vi "LS218_READ_KELVIN.vi"(3 "entrée d'erreur (pas d'erreur)":errorcluster, 4 "numéro voie":i32, 5 "Refnum VISA en entrée":refnum<visa-resource-name>) -> (0 "sortie d'erreur":errorcluster, 1 "T_Kelvin":dbl, 2 "Nom de ressource VISA en sortie":refnum<visa-resource-name>)   [LabVIEW 2016]
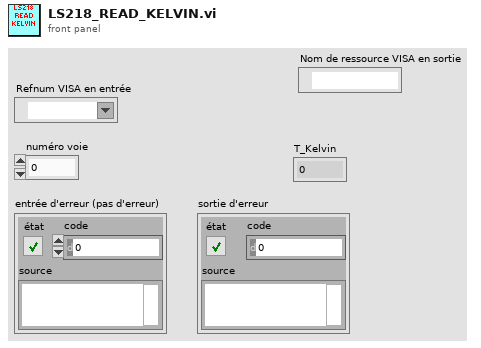
[diagram p1: front panel]
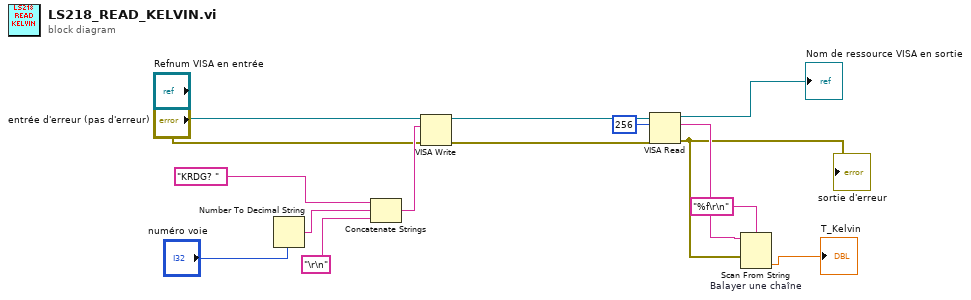
[diagram p0: block diagram]
diagram:
  n1 = Number To Decimal String(number="numéro voie") -> (decimal integer string=w15:string)  [unwired: 1 in]
  n2 = Concatenate Strings("KRDG? " ("chaîne"), w15, "\r\n" ("chaîne")) -> (w13:string)
  n3 = VISA Write(VISA resource name="Refnum VISA en entrée", write buffer=w13, error in (no error)="entrée d'erreur (pas d'erreur)") -> (VISA resource name out=w8:refnum<visa-resource-name>, error out=w9:errorcluster)  [unwired: 1 out]
  n4 = VISA Read(VISA resource name=w8, byte count=u32 256 ("nombre d'octets"), error in (no error)=w9) -> (VISA resource name out=→"Nom de ressource VISA en sortie":refnum<visa-resource-name>, read buffer=w4:string, error out=w3:errorcluster)  [unwired: 1 out]
  "sortie d'erreur" <- w3
  n5 = Scan From String "Balayer une chaîne"(format string="%f\r\n" ("chaîne de format"), input string=w4, error in=w3) -> (output 1=→"T_Kelvin":dbl)  [unwired: 2 in, 3 out]
